vi "test Create New Import Aliases.vi"(8 "error in (no error)":errorcluster, 11 "TestCase in":refnum<class "Routing and Faulting Import Unit Tests.lvclass">) -> (0 "error out":errorcluster, 3 "TestCase out":refnum<class "Routing and Faulting Import Unit Tests.lvclass">)   [LabVIEW 2017, in "Routing and Faulting Import Unit Tests.lvclass"]
uses:
  Routing and Faulting Import Unit Tests.lvclass
  Shared/Alias Mapping.ctl
  <vilib>/addons/_JKI Toolkits/VI Tester/TestCase.llb/TestCase.lvclass
  <vilib>/NI/NI VeriStand Custom Device Import and Export Tool/ImportExport.lvlib
  Scripting/Routing and Faulting Scripting.lvlib
  Shared/Routing and Faulting Shared.lvlib
  C:/Program Files (x86)/National Instruments/LabVIEW 2017/vi.lib/addons/_JKI Toolkits/VI Tester/TestCase.llb/TestCase.lvclass
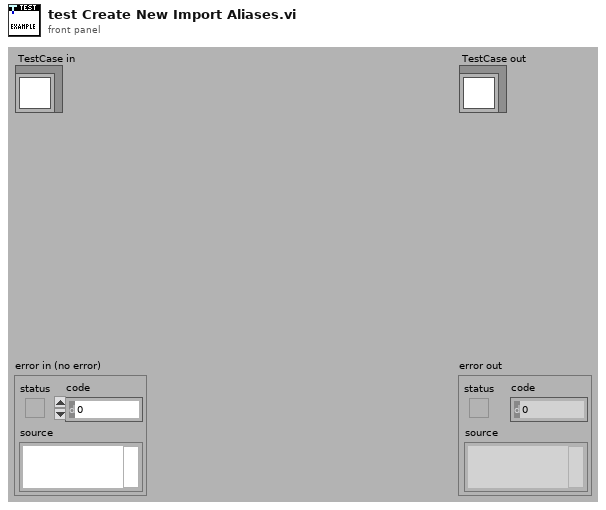
[diagram p1: front panel]
types:
  T1 = typedef "Routing and Faulting Shared.lvlib/Alias Mapping.ctl" = cluster{"Endpoint":string, "Alias":string}
  T2 = typedef "Custom Device API.lvlib/Custom Device Item Ref.ctl" = u64
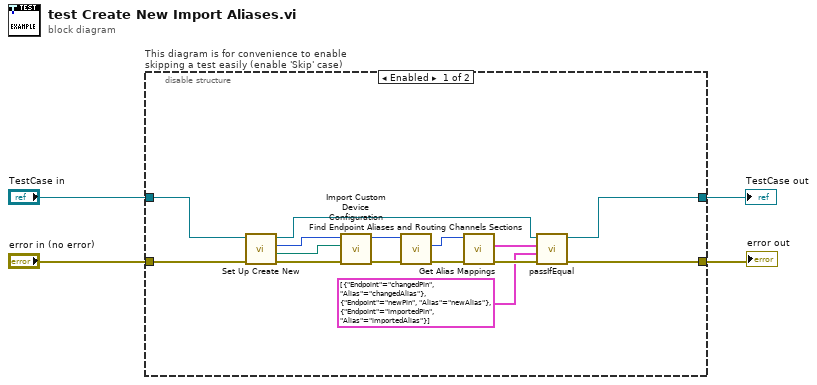
[diagram p0: block diagram]
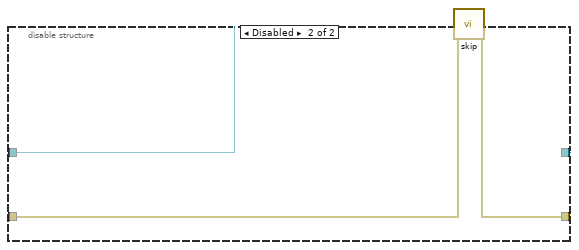
[diagram p2: hidden frame]
diagram:
  n1 = disable-structure "This diagram is for convenience to enable skipping a test easily (enable 'Skip' case)" shown="Enabled" {
    disable-tunnel: "TestCase in" -> [w10 w23]
    disable-tunnel: [w9 w21] -> w1
    disable-tunnel: [w8 w22] -> w3
    disable-tunnel: "error in (no error)" -> [w15 w20]
    frame Enabled {
      n2 = call "Set Up Create New.vi"("error in (no error)"=w15, "Test Case in"=w10) -> ("error out"=w14:errorcluster, "Import Path"=w12:path, "Routing and Faulting Custom Device Ref"=w13:T2, "Test Case out"=w7:refnum<class "Routing and Faulting Import Unit Tests.lvclass">)  [unwired: 6 in]
      n3 = call <vilib>:"Import Custom Device Configuration.vi"("error in (no error)"=w14, "Path"=w12, "NodeID"=w13) -> ("error out"=w18:errorcluster, "NodeID out"=w19:u64)  [unwired: 6 in, 1 out]
      n4 = call "Find Endpoint Aliases and Routing Channels Sections.vi"("error in (no error)"=w18, "Routing and Faulting Custom Device Ref in"=w19) -> ("error out"=w17:errorcluster, "Endpoint Aliases Ref"=w16:T2)  [unwired: 6 in, 2 out]
      n5 = call "Get Alias Mappings.vi"("error in (no error)"=w17, "Endpoint Aliases Ref in"=w16) -> ("error out"=w11:errorcluster, "Alias Mappings"=w5:T1[])  [unwired: 7 in, 1 out]
      n6 = call-dynamic "passIfEqual.vi"("error in (no error)"=w11, "y"=T1[] [{"Endpoint"="changedPin", "Alias"="changedAlias"}, {"Endpoint"="newPin", "Alias"="newAlias"}, {"Endpoint"="importedPin", "Alias"="importedAlias"}] ("Alias Mappings"), "x"=w5, "TestCase in"=w7) -> ("error out"=w8:errorcluster, "TestCase out"=w9:refnum<class "Routing and Faulting Import Unit Tests.lvclass">)  [unwired: 6 in]
    }
    frame Disabled {
      # "skip test result while test is under development"
      n7 = call <vilib>:"skip.vi"("error in (no error)"=w20, "TestCase in"=w23) -> ("error out"=w22:errorcluster, "TestCase out"=w21:refnum<class "Routing and Faulting Import Unit Tests.lvclass">)  [unwired: 8 in]
    }
  }
  "error out" <- w3
  "TestCase out" <- w1
